vi "Load Plugins.vi"(8 "Error In":errorcluster, 10 "Folder Path":path, 11 "Factory Plugin Framework in":refnum<class "Factory Plugin Framework.lvclass">=refnum) -> (0 "Error Out":errorcluster, 3 "Factory Plugin Framework out":refnum<class "Factory Plugin Framework.lvclass">)   [LabVIEW 2018, in "Factory Plugin Framework.lvlib" / "Factory Plugin Framework.lvclass"]
uses:
  Factory Plugin Framework.lvclass
  <vilib>/Utility/LVLibp/NI_PackedLibraryUtility.lvlib
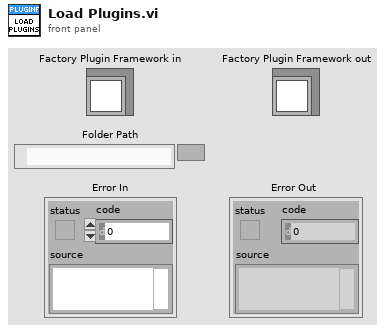
[diagram p1: front panel]
types:
  T1 = cluster{"Plugin Name":string, "Plugin Object":refnum<class>}
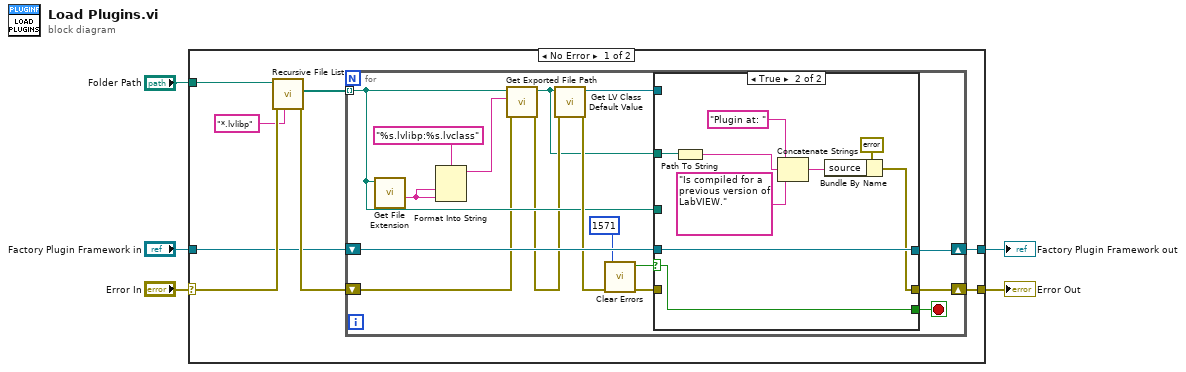
[diagram p0: block diagram]
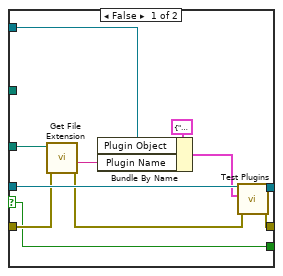
[diagram p2: hidden frame]
diagram:
  n1 = case shown="No Error" "Error In" {
    selector: "Error In" -> [w12 w51]
    tunnel: [w8 w51] -> w4
    tunnel: [w6 w50] -> w2
    tunnel: "Factory Plugin Framework in" -> [w7 w50]
    tunnel: "Folder Path" -> [w13 _]
    frame No Error {
      n2 = call <vilib>:"Recursive File List.vi"("pattern"="*.lvlibp", "error in (no error)"=w12, "Folder Path"=w13) -> ("error out"=w10:errorcluster, "All Files in Dir"=w9:path[])  [unwired: 4 in, 3 out]
      n3 = for {
        shift-right: [w29] -> w8
        shift-left: w10 -> [w20]
        tunnel: w9 -> [w22] mode=indexing
        shift-right: [w28] -> w6
        shift-left: w7 -> [w27]
        stop <- w14 stop-if-true
        n4 = call <vilib>:"Get File Extension.vi"("file"=w22) -> ("filename without extension"=w24:string)  [unwired: 6 in, 4 out]
        n5 = Format Into String(format string="%s.lvlibp:%s.lvclass", w24, w24) -> (resulting string=w21:string)  [unwired: 2 in, 1 out]
        n6 = call <vilib>:"Get Exported File Path.vi"("error in (no error)"=w20, "qualified name"=w21, "packed library path"=w22) -> ("error out"=w19:errorcluster, "path"=w15:path)  [unwired: 7 in]
        n7 = call <vilib>:"Get LV Class Default Value.vi"("error in (no error)"=w19, "class path"=w15) -> ("error out"=w26:errorcluster, "object"=w25:refnum<class>)  [unwired: 8 in]
        n8 = call <vilib>:"Clear Errors.vi"("error in (no error)"=w26, "specific error code to clear (0: all)"=1571) -> ("error out"=w18:errorcluster, "specific error cleared?"=w16:bool)  [unwired: 4 in]
        n9 = case shown="True" w16 {
          selector: w16 -> [w30 w41]
          tunnel: [w40 w47] -> w29
          tunnel: [w39 w49] -> w28
          tunnel: w27 -> [w38 w49]
          tunnel: w25 -> [w33 _]
          tunnel: w22 -> [w32 _]
          tunnel: w18 -> [w31 _]
          tunnel: w15 -> [_ w46]
          tunnel: [w30 w41] -> w14
          frame False {
            n10 = call <vilib>:"Get File Extension.vi"("error in (no error)"=w31, "file"=w32) -> ("error out"=w37:errorcluster, "filename without extension"=w34:string)  [unwired: 5 in, 3 out]
            n11 = Bundle By Name(cluster=T1 {"Plugin Name"="", "Plugin Object"=refnum} ("Plugin Data"), "Plugin Object"=w33, "Plugin Name"=w34) -> (w35:T1)
            n12 = call "Test Plugins.vi"("Error In"=w37, "Plugin Data"=w35, "Factory Plugin Framework in"=w38) -> ("Error Out"=w40:errorcluster, "Factory Plugin Framework out"=w39:refnum<class "Factory Plugin Framework.lvclass">)  [unwired: 7 in]
          }
          frame True {
            n13 = Path To String(path=w46) -> (string=w44:string)
            n14 = Concatenate Strings("Plugin at: ", w44, "Is compiled for a previous version of LabVIEW.") -> (w42:string)
            n15 = Bundle By Name(cluster=errorcluster {"status"=TRUE, "code"=1571, "source"=""} ("Error Out"), "source"=w42) -> (w47:errorcluster)
          }
        }
      }
    }
    frame Error {
    }
  }
  "Error Out" <- w4
  "Factory Plugin Framework out" <- w2
